vi "SVFA Zoom FFT Spectrum (Mag-Phase) (1 Ch).vi"(0 "scaled signal [EU]":waveform(dbl)={"t0"=timestamp(0 s since 1904-01-01), "dt"=1e-05, "Y"=[]}, 3 "zoom settings":T2={"frequency range"={"start frequency"=1000.0, "stop frequency"=2000.0}, "window"=1, "number of lines"=400, "% overlap"=0.0} {"% overlap" min=0.0 format="%.2f"; "number of lines" min=2; "window" items=["None ", "Hanning", "Hamming", "Blackman-Harris", "Exact Blackman", "Blackman", "Flat Top", "4 Term B-Harris ", "7 Term B-Harris", "Low Sidelobe"]; "frequency range"."stop frequency" min=0.0 format="%.2f"; "frequency range"."start frequency" min=0.0 format="%.2f"}, 4 "view":T1={"dB On (T)"=TRUE, "unwrap phase (F)"=FALSE, "convert to degree (T)"=TRUE}, 5 "error in (no error)":errorcluster, 7 "averaging parameters":T9={"averaging mode"=enum."No averaging", "weighting mode"=enum."Exponential", "number of averages"=10, "linear mode"=enum."One shot"} {"number of averages" min=1 step=1}, 9 "restart averaging (F)":bool) -> (11 "averaging done":bool, 12 "new spectrum available":bool, 13 "averages completed":dbl, 14 "magnitude [dB EU]":cluster{"f0":dbl, "df":dbl, "magnitude":dbl[]} {"magnitude" format="%.2p"; "df" format="%.2p"; "f0" format="%.2p"}, 15 "magnitude unit label":string, 16 "phase [degrees]":cluster{"f0":dbl, "df":dbl, "phase":dbl[]} {"phase" format="%.2p"; "df" format="%.2p"; "f0" format="%.2p"}, 17 "phase unit label":string, 18 "spectrum info":T3={"channel name"="", "description"="", "x-axis units"=0, "spectral info"={"spectrum type"=enum."Power [Magnitude^2]", "linear/dB"=enum."linear", "window"=0, "window size"=0, "FFT size"=0}, "engineering units"=0, "custom label"="", "dB reference [EU]"=0.0, "peak units"=enum."rms", "weighting filter"=0, "spectral density?"=FALSE, "unit label"="", "spectrum skewed?"=FALSE, "complimentary spectrum units"=enum."none"} {"x-axis units" items=["Time (s)"=0, "Frequency-CB (Hz)"=1, "Frequency-CPB (Hz)"=1248, "Frequency-Arbitrary (Hz)"=2357, "Quefrency (s)"=2, "Revolutions (rev)"=3, "Order"=4, "Speed (RPM)"=11, "Speed (rad/s)"=21, "Index"=65535]; "weighting filter" items=["Linear", "A-weighting", "B-weighting", "C-weighting", "ITU-R 468-4", "Dolby", "CCITT", "C-message", "Wb", "Wc", "Wd", "We", "Wf", "Wh", "Wj", "Wk", "Wm", "AES17 20 kHz lowpass", "AES17 40 kHz lowpass", "AES17 20 kHz highpass", "AES17 40 kHz highpass"]; "dB reference [EU]" format="%.2f"; "engineering units" items=["custom..."=0, "V"=1, "A"=21, "C"=30, "pC"=31, "s"=32, "-"=29, "Pa"=2, "N"=20, "g"=3, "m/s^2"=4, "m/s"=5, "m"=6, "mm/s"=12, "mm"=13, "micron/s"=14, "micron"=15, "in/s^2"=7, "in/s"=8, "in"=9, "mil/s"=10, "mil"=11, "rad/s^2"=16, "rad/s"=17, "rad"=18, "deg/s^2"=26, "deg/s"=27, "deg"=28, "RPM"=22, "cycle/s^2"=23, "Hz"=24, "cycle"=25, "strain"=19]; "spectral info"."window" items=["None "=0, "Hanning"=1, "Hamming"=2, "Blackman-Harris"=3, "Exact Blackman"=4, "Blackman"=5, "Flat Top"=6, "4 Term B-Harris "=7, "7 Term B-Harris"=8, "Low Sidelobe"=9, "Force - Exponential"=10, "Gaussian"=62]}, 19 "error out":errorcluster)   [LabVIEW 2017]
doc: "Computes the zoom FFT spectrum of <B>scaled signal [EU]</B> and <B>zoom settings</B>. Zoom FFT results are returned in magnitude and phase. Data accumulates each time this VI is called. However, it returns a new spectrum only when sufficient data accumulates. Indicators and subsequent processing should only be called when <B>new spectrum available</B> is TRUE. Wire data to the <B>scaled signal [EU]</B> input to determine the polymorphic instance to use or manually select the instance."
uses:
  <vilib>/addons/_NISVFA/_Shared subVIs/Controls/svc_Spectrum Info.ctl
  <vilib>/addons/_NISVFA/_Shared subVIs/Controls/svc_X-Axis Units.ctl
  <vilib>/addons/_NISVFA/_Shared subVIs/Controls/svc_Spectrum Type.ctl
  <vilib>/addons/_NISVFA/_Shared subVIs/Controls/svc_Engineering Units Text Ring.ctl
  <vilib>/addons/_NISVFA/_Shared subVIs/Controls/svc_Weighting Filter Text Ring.ctl
  <vilib>/addons/_NISVFA/_Shared subVIs/Controls/svc_Complimentary Spectrum Units.ctl
  <vilib>/addons/_NISVFA/_Shared subVIs/Common/svc_Get SV Channel Info.vi
  <vilib>/addons/_NISVFA/_Shared subVIs/Common/svc_Spectrum Units.vi
  <vilib>/addons/_NISVFA/_Shared subVIs/Spectrum Averaging/svfa_Reset Averaging State Info.vi
  <vilib>/addons/_NISVFA/_Shared subVIs/Spectrum Averaging/svfa_Average Array with Avg Checks (complex) No State.vi
  <vilib>/addons/_NISVFA/_Shared subVIs/Common/svc_Complex to Mag2 Array.vi
  <vilib>/addons/_NISVFA/_Shared subVIs/Spectrum Averaging/svfa_Average Array with Avg Checks (real) No State.vi
  <vilib>/addons/_NISVFA/_Shared subVIs/Spectrum Averaging/svfa_Average Array (complex) No State.vi
  <vilib>/addons/_NISVFA/_Shared subVIs/Spectrum Averaging/svfa_Average Array (real) No State.vi
  <vilib>/addons/_NISVFA/_Shared subVIs/Spectrum Averaging/svfa_No Average Array (complex).vi
  <vilib>/addons/_NISVFA/_Shared subVIs/Spectrum Averaging/svfa_Average Array (complex).vi
  <vilib>/addons/_NISVFA/_Shared subVIs/Spectrum Averaging/svfa_No Average Array (real).vi
  <vilib>/addons/_NISVFA/_Shared subVIs/Spectrum Averaging/svfa_Average Array (real).vi
  <vilib>/addons/_NISVFA/_Shared subVIs/Spectrum Averaging/svfa_Peak Hold Array.vi
  <vilib>/addons/_NISVFA/_Shared subVIs/Common/svc_Get Weighting Enum and Labels.vi
  <vilib>/addons/_NISVFA/_Shared subVIs/Common/svc_Unit Label Lexical Class.vi
  <vilib>/addons/_NISVFA/_Shared subVIs/Common/svc_Engineering Units to Unit Label.vi
  <vilib>/addons/_NISVFA/_Shared subVIs/Common/svc_Format Value (DBL).vi
  <vilib>/addons/_NISVFA/_Shared subVIs/Common/svc_Channel Info to Spectrum Info.vi
  <vilib>/addons/_NISVFA/_Shared subVIs/Common/svc_Unit Label to Engineering Units.vi
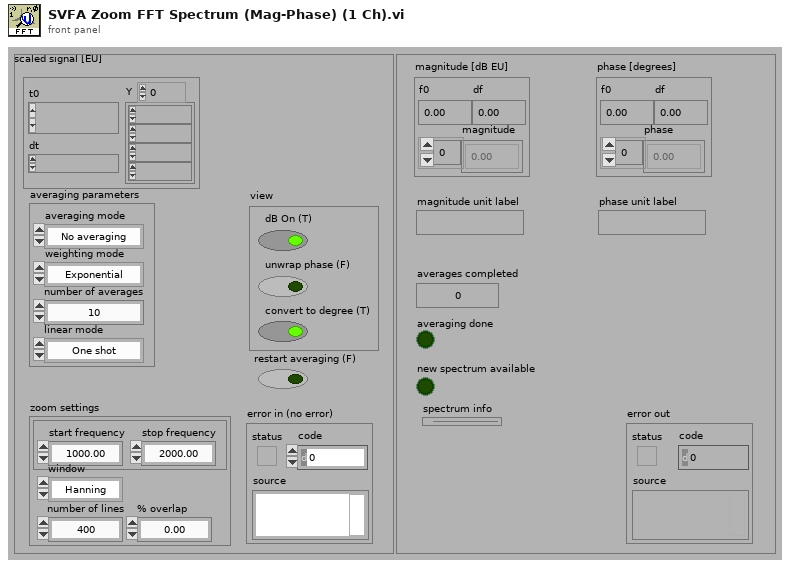
[diagram p1: front panel]
types:
  T1 = cluster{"dB On (T)":bool, "unwrap phase (F)":bool, "convert to degree (T)":bool}
  T2 = cluster{"frequency range":cluster{"start frequency":dbl, "stop frequency":dbl}, "window":u16, "number of lines":i32, "% overlap":dbl}
  T3 = typedef "svc_Spectrum Info.ctl" = cluster{"channel name":string, "description":string, "x-axis units":T4, "spectral info":cluster{"spectrum type":T5, "linear/dB":enum16{"linear", "dB"}, "window":u16, "window size":i32, "FFT size":i32}, "engineering units":T6, "custom label":string, "dB reference [EU]":dbl, "peak units":enum16{"rms", "peak", "peak-peak"}, "weighting filter":T7, "spectral density?":bool, "unit label":string, "spectrum skewed?":bool, "complimentary spectrum units":T8}
  T4 = typedef "svc_X-Axis Units.ctl" = u16
  T5 = typedef "svc_Spectrum Type.ctl" = enum16{"FFT Spectrum [complex]", "Amplitude [Magnitude]", "Power [Magnitude^2]", "Cross Spectrum [complex]", "Frequency Response [Complex]"}
  T6 = typedef "svc_Engineering Units Text Ring.ctl" = u16
  T7 = typedef "svc_Weighting Filter Text Ring.ctl" = u16
  T8 = typedef "svc_Complimentary Spectrum Units.ctl" = enum16{"none", "radians", "degrees", "cycles", "imaginary"}
  T9 = cluster{"averaging mode":enum16{"No averaging", "Vector averaging", "RMS averaging", "Peak hold"}, "weighting mode":enum16{"Linear", "Exponential"}, "number of averages":u32, "linear mode":enum16{"One shot", "Auto restart"}}
  T10 = enum16{"Restart processing", "Continue processing", "Skip processing"}
  T11 = enum16{"No averaging", "Vector averaging", "RMS averaging", "Peak hold"}
  T12 = cluster{"zoom settings":cluster{"center frequency":dbl, "zoom":i32, "trim":dbl}, "FFT settings":cluster{"window":enum16{"None ", "Hanning", "Hamming", "Blackman-Harris", "Exact Blackman", "Blackman", "Flat Top", "4 Term B-Harris ", "7 Term B-Harris", "Low Sidelobe"}, "window size":i32, "FFT size":i32, "%overlap":dbl}}
  T13 = cluster{"complex FFT":cdb[], "real FFT":dbl[], "f0":dbl, "df":dbl, "averages completed":dbl, "averaging parameters":cluster{"averaging mode":enum16{"No averaging", "Vector averaging", "RMS averaging", "Peak hold"}, "weighting mode":enum16{"Linear", "Exponential"}, "number of averages":u32, "linear mode":enum16{"One shot", "Auto restart"}}}
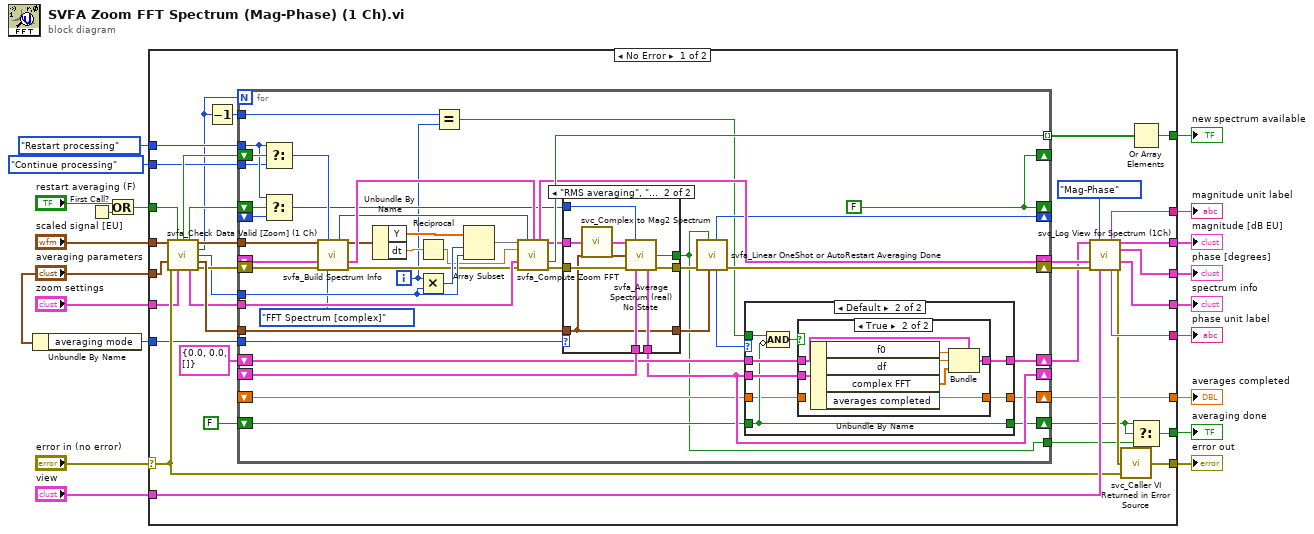
[diagram p0: block diagram]
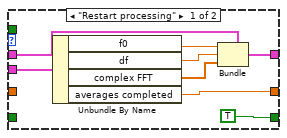
[diagram p2: hidden frame]
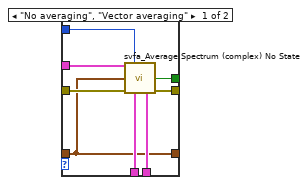
[diagram p4: hidden frame]
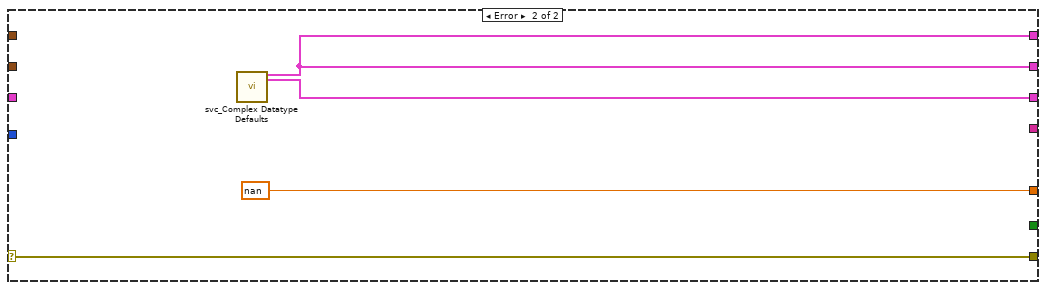
[diagram p5: hidden frame]
diagram:
  n1 = Unbundle By Name("averaging parameters") -> ("averaging mode"=w1:T11)
  n2 = First Call?() -> (First Call?: T/F=w7:bool)
  n3 = Or(x="restart averaging (F)", y=w7) -> (x .or. y?=w5:bool)
  n4 = case shown="No Error" "error in (no error)" {
    selector: "error in (no error)" -> [w48 w148]
    tunnel: w5 -> [w38 _]
    tunnel: [w28 nan ("Averaged So-far")] -> w20
    tunnel: [w27 _] -> w19
    tunnel: [w49 w148] -> w18
    tunnel: "averaging parameters" -> [w56 _]
    tunnel: "zoom settings" -> [w44 _]
    tunnel: "scaled signal [EU]" -> [w57 _]
    tunnel: [w50 w145] -> w8
    tunnel: [w54 _] -> w14
    tunnel: [w22 _] -> w13
    tunnel: [w52 w146] -> w12
    tunnel: [w53 w146] -> w11
    tunnel: [w26 _] -> w10
    tunnel: "view" -> [w55 _]
    tunnel: T10."Restart processing" ("processing control") -> [w36 _]
    tunnel: T10."Continue processing" ("processing control") -> [w35 _]
    tunnel: w1 -> [w34 _]
    frame No Error {
      n5 = call <vilib>:"svfa_Check Data Valid [Zoom] (1 Ch).vi"("signal [V]"=w57, "restart averaging (F)"=w38, "averaging parameters"=w56, "error in (no error)"=w48, "zoom settings"=w44) -> ("reset processing"=w37:bool, "restart averaging"=w42:bool, "dup signal [V]"=w47:waveform(dbl), "iterations"=w33:i32, "maximum block size"=w39:i32, "dup averaging parameters"=w46:T9, "zoom FFT settings"=w43:T12, "error out"=w45:errorcluster)  [unwired: 3 in]
      n6 = Decrement(x=w33) -> (x-1=w32:i32)
      n7 = for {
        N: w33 -> [_]
        shift-left: _ -> [w98]
        shift-right: [w65] -> _
        tunnel: [w99] -> w40 mode=indexing
        tunnel: w43 -> [w100]
        tunnel: [w58] -> w25
        shift-right: [w97] -> w29
        shift-left: _ -> [w96]
        shift-right: [w68] -> _
        shift-left: _ -> [w92]
        tunnel: w46 -> [w95]
        tunnel: w36 -> [w76]
        tunnel: w47 -> [w101]
        shift-right: [w59] -> _
        shift-left: w42 -> [w93]
        tunnel: w39 -> [w91]
        shift-right: [w59] -> _
        shift-left: w37 -> [w77]
        tunnel: w35 -> [w75]
        tunnel: w34 -> [w72]
        tunnel: w32 -> [w70]
        shift-right: [w64] -> w23
        shift-left: cluster{"f0":dbl, "df":dbl, "real FFT":cdb[]} {"f0"=0.0, "df"=0.0, "real FFT"=[]} -> [w66]
        shift-right: [w63] -> w28
        shift-left: _ -> [w62]
        shift-right: [w61] -> w24
        shift-left: FALSE ("restart averaging") -> [w60]
        shift-right: [w102] -> w41
        shift-left: w45 -> [w94]
        i -> [w69]
        w59 = FALSE ("restart averaging")
        n8 = Select(t=w76, s=w77, f=w75) -> (s? t:f=w74:T10)
        n9 = Select(t=w76, s=w93, f=w92) -> (s? t:f=w73:T10)
        n10 = call <vilib>:"svfa_Build Spectrum Info.vi"("scaled signal [EU]"=w101, "processing control"=w74, "spectrum info in"=w96, "error in (no error)"=w94, "spectrum type"=svc_Spectrum_Type."FFT Spectrum [complex]") -> ("dup processing control"=w79:T10, "dup scaled signal [EU]"=w82:waveform(dbl), "spectrum info out"=w87:T3, "error out"=w80:errorcluster)  [unwired: 7 in]
        n11 = Unbundle By Name ("Get Waveform Components")(w82) -> ("Y"=w88:dbl[], "dt"=w86:dbl)
        n12 = Reciprocal(x=w86) -> (1/x=w81:dbl)
        n13 = Multiply(x=w69, y=w91) -> (x*y=w90:i32)
        n14 = Equal?(x=w70, y=w69) -> (x = y?=w67:bool)
        n15 = Array Subset(array=w88, index=w90, length=w91) -> (w78:dbl[])
        n16 = call <vilib>:"svfa_Compute Zoom FFT.vi"("x"=w78, "processing control"=w79, "spectrum info"=w87, "fs"=w81, "zoom FFT settings"=w100, "error in (no error)"=w80) -> ("spectrum info out"=w97:T3, "FFT spectrum"=w84:cluster{"f0":dbl, "df":dbl, "spectrum":cdb[]}, "spectrum ready"=w99:bool, "error out"=w83:errorcluster)  [unwired: 5 in, 1 out]
        n17 = case shown="\"RMS averaging\", \"Peak hold\"" w72 {
          tunnel: w95 -> [w128 w136]
          tunnel: [w133 w139] -> w89
          tunnel: [w132 w143] -> w58
          tunnel: w84 -> [w135 w140]
          tunnel: w83 -> [w134 w144]
          tunnel: w73 -> [w131 w141]
          tunnel: [w130 w137] -> w65
          tunnel: w98 -> [w129 w138]
          tunnel: [w128 w136] -> w71
          frame "No averaging", "Vector averaging" {
            n18 = call <vilib>:"svfa_Average Spectrum (complex) No State.vi"("spectrum"=w135, "processing control"=w131, "averaging parameters"=w128, "error in (no error)"=w134, "averaging state info in"=w129) -> ("averaging done"=w132:bool, "averaging state info out"=w130:T13, "error out"=w133:errorcluster)  [unwired: 5 in, 3 out]
          }
          frame "RMS averaging", "Peak hold" {
            n19 = call <vilib>:"svc_Complex to Mag2 Spectrum.vi"("complex spectrum"=w140) -> ("power spectrum"=w142:cluster{"f0":dbl, "df":dbl, "spectrum":dbl[]})  [unwired: 4 in]
            n20 = call <vilib>:"svfa_Average Spectrum (real) No State.vi"("spectrum"=w142, "processing control"=w141, "averaging parameters"=w136, "error in (no error)"=w144, "averaging state info in"=w138) -> ("averaging done"=w143:bool, "averaging state info out"=w137:T13, "error out"=w139:errorcluster)  [unwired: 5 in, 3 out]
          }
        }
        n21 = call <vilib>:"svfa_Linear OneShot or AutoRestart Averaging Done.vi"("averaging parameters"=w71, "averaging done"=w58, "error in (no error)"=w89) -> ("error out"=w102:errorcluster, "processing control"=w68:T10)  [unwired: 7 in]
        n22 = case shown="Default" w68 {
          tunnel: w65 -> [w107 w118]
          tunnel: [TRUE ("restart averaging") w113] -> w61
          tunnel: [w105 w117] -> w64
          tunnel: w60 -> [_ w113]
          tunnel: w67 -> [_ w116]
          tunnel: w66 -> [w104 w115]
          tunnel: [w103 w112] -> w63
          tunnel: w62 -> [_ w111]
          frame "Restart processing" {
            n23 = Unbundle By Name(w107) -> ("f0"=w110:dbl, "df"=w109:dbl, "complex FFT"=w108:cdb[], "averages completed"=w103:dbl)
            n24 = Bundle(cluster=w104, "f0"=w110, "df"=w109, "real FFT"=w108) -> (w105:cluster{"f0":dbl, "df":dbl, "real FFT":cdb[]})
          }
          frame Default {
            n25 = Compound Arithmetic op=AND(w116, invert w113) -> (w114:bool)
            n26 = case shown="True" w114 {
              tunnel: w118 -> [_ w124]
              tunnel: [w120 w123] -> w117
              tunnel: w115 -> [w120 w122]
              tunnel: [w119 w121] -> w112
              tunnel: w111 -> [w119 _]
              frame False {
              }
              frame True {
                n27 = Unbundle By Name(w124) -> ("f0"=w127:dbl, "df"=w126:dbl, "complex FFT"=w125:cdb[], "averages completed"=w121:dbl)
                n28 = Bundle(cluster=w122, "f0"=w127, "df"=w126, "real FFT"=w125) -> (w123:cluster{"f0":dbl, "df":dbl, "real FFT":cdb[]})
              }
            }
          }
        }
      }
      n29 = call <vilib>:"svc_Log View for Spectrum (1Ch).vi"("complex spectrum"=w23, "View"=enum16{"Mag-Phase", "Real-Imaginary"}."Mag-Phase", "spectrum info in"=w29, "error in (no error)"=w41, "view"=w55) -> ("unit label [mag or real]"=w22:string, "magnitude or real"=w53:cluster{"f0":dbl, "df":dbl, dbl[]}, "phase or imag"=w52:cluster{"f0":dbl, "df":dbl, dbl[]}, "spectrum info out"=w50:T3, "unit label [phase or imag]"=w54:string, "error out"=w51:errorcluster)  [unwired: 5 in]
      n30 = call <vilib>:"svc_Caller VI Returned in Error Source.vi"("warning input to caller"=w48, "error in (no error)"=w51) -> ("error out"=w49:errorcluster)  [unwired: 3 in]
      n31 = Or Array Elements(Boolean array=w40) -> (logical OR=w27:bool)
      n32 = Select(t=w24, s=w24, f=w25) -> (s? t:f=w26:bool)
    }
    frame Error {
      n33 = call <vilib>:"svc_Complex Datatype Defaults.vi"() -> ("empty spectrum"=w146:cluster{"f0":dbl, "df":dbl, "magnitude":dbl[]}, "dead spectrum info"=w145:T3)  [unwired: 11 in, 7 out]
    }
  }
  "averages completed" <- w20
  "new spectrum available" <- w19
  "error out" <- w18
  "spectrum info" <- w8
  "magnitude unit label" <- w13
  "phase unit label" <- w14
  "magnitude [dB EU]" <- w11
  "phase [degrees]" <- w12
  "averaging done" <- w10
